vi "StanfordResSysDG645DelayGenerator.vi"() -> ()   [LabVIEW 2020]
uses:
  lib/Hardware/TextControlledInstrumIOQueuePacket.ctl
  lib/Hardware/TextControlledInstrum/TextControlledInstrumControlToCommandMulti.vi
panel:
  in  "SHOW LOG":bool
  in  "BURST":T1 {"Period (s)" format="%#_6p"; "Delay (s)" format="%#_6p"}
  in  "ErrChk":bool
  in  "Enable":bool
  out "ID":string
  in  "TRIGGER":T2 {"Level (V)" format="%#_6p"; "Rate (Hz)" format="%#_6p"; "Source" items=["Internal", "Ext Rising Edge", "Ext Falling Edge", "Single Shot Ext Rising", "Single Shot Ext Falling", "Single Shot", "Line"]}
  out "LOG":string
  in  "T0T1":T3 {"Delay T1" format="%#_6p"; "Delay T0" format="%#_6p"}
  in  "GH":T4 {"Delay H" format="%#_6p"; "Delay G" format="%#_6p"}
  in  "EF":T5 {"Delay F" format="%#_6p"; "Delay E" format="%#_6p"}
  in  "CD":T6 {"Delay D" format="%#_6p"; "Delay C" format="%#_6p"}
  in  "AB":T7 {"Delay B" format="%#_6p"; "Delay A" format="%#_6p"}
  in  "VISA resource name":refnum<visa-resource-name>
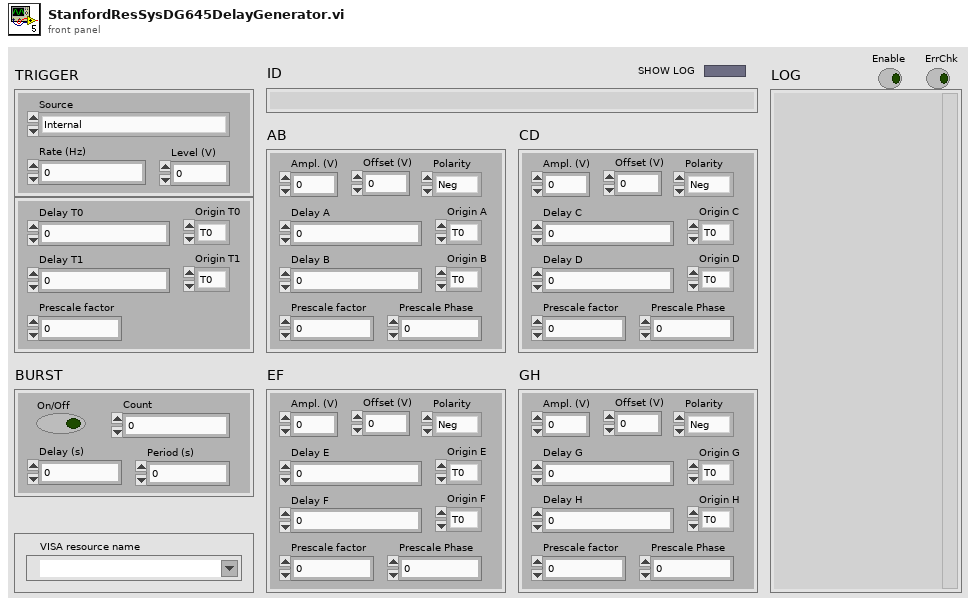
[diagram p1: front panel]
types:
  T1 = cluster{"On/Off":bool, "Count":u32, "Delay (s)":ext, "Period (s)":ext}
  T2 = cluster{"Source":u16, "Rate (Hz)":ext, "Level (V)":ext}
  T3 = cluster{"DLAY T0":string, "DLAY T1":string, "Delay T0":ext, "Origin T0":enum16{"T0", "T1", "A", "B", "C", "D", "E", "F", "G", "H"}, "Delay T1":ext, "Origin T1":enum16{"T0", "T1", "A", "B", "C", "D", "E", "F", "G", "H"}, "Prescale factor":u32}
  T4 = cluster{"Ampl. (V)":dbl, "Offset (V)":dbl, "Polarity":enum16{"Neg", "Pos"}, "DLAY G":string, "DLAY H":string, "Delay G":ext, "Origin G":enum16{"T0", "T1", "A", "B", "C", "D", "E", "F", "G", "H"}, "Delay H":ext, "Origin H":enum16{"T0", "T1", "A", "B", "C", "D", "E", "F", "G", "H"}, "Prescale factor":u32, "Prescale Phase":u32}
  T5 = cluster{"Ampl. (V)":dbl, "Offset (V)":dbl, "Polarity":enum16{"Neg", "Pos"}, "DLAY E":string, "DLAY F":string, "Delay E":ext, "Origin E":enum16{"T0", "T1", "A", "B", "C", "D", "E", "F", "G", "H"}, "Delay F":ext, "Origin F":enum16{"T0", "T1", "A", "B", "C", "D", "E", "F", "G", "H"}, "Prescale factor":u32, "Prescale Phase":u32}
  T6 = cluster{"Ampl. (V)":dbl, "Offset (V)":dbl, "Polarity":enum16{"Neg", "Pos"}, "DLAY C":string, "DLAY D":string, "Delay C":ext, "Origin C":enum16{"T0", "T1", "A", "B", "C", "D", "E", "F", "G", "H"}, "Delay D":ext, "Origin D":enum16{"T0", "T1", "A", "B", "C", "D", "E", "F", "G", "H"}, "Prescale factor":u32, "Prescale Phase":u32}
  T7 = cluster{"Ampl. (V)":dbl, "Offset (V)":dbl, "Polarity":enum16{"Neg", "Pos"}, "DLAY A":string, "DLAY B":string, "Delay A":ext, "Origin A":enum16{"T0", "T1", "A", "B", "C", "D", "E", "F", "G", "H"}, "Delay B":ext, "Origin B":enum16{"T0", "T1", "A", "B", "C", "D", "E", "F", "G", "H"}, "Prescale factor":u32, "Prescale Phase":u32}
  T8 = typedef "TextControlledInstrumIOQueuePacket.ctl" = cluster{"Operation":enum16{"read", "write", "reserved2", "reserved3", "reserved4", "reserved5", "reserved6", "reserved7"}, "Data":string, "Queue":refnum<queue>}
  T9 = enum16{"read", "write", "reserved2", "reserved3", "reserved4", "reserved5", "reserved6", "reserved7"}
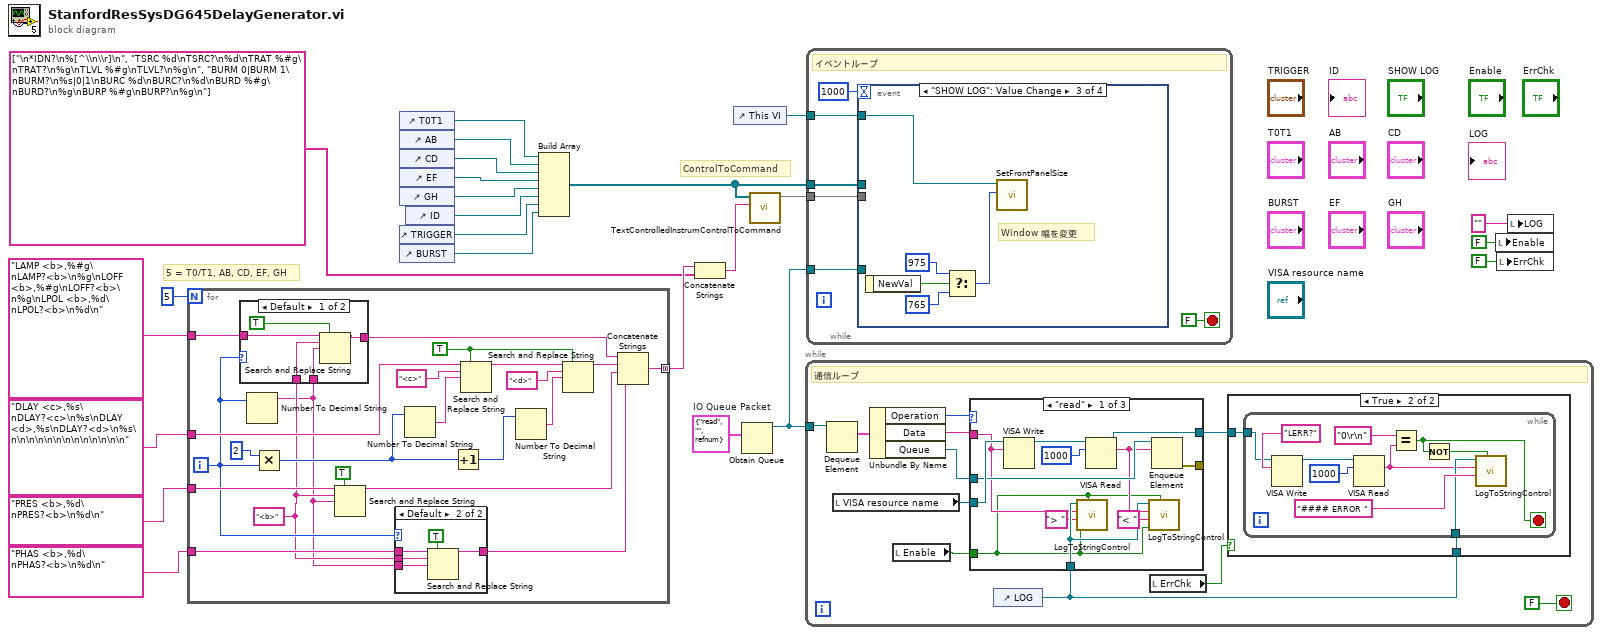
[diagram p0: block diagram]
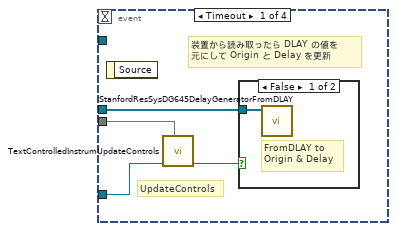
[diagram p4: hidden frame]
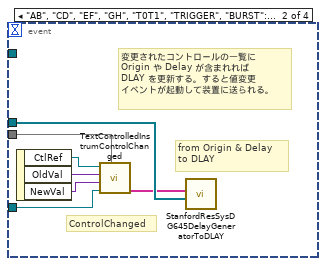
[diagram p6: hidden frame]
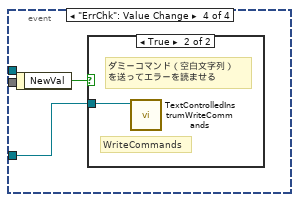
[diagram p7: hidden frame]
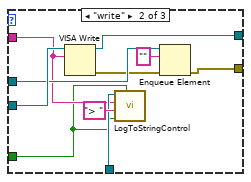
[diagram p9: hidden frame]
diagram:
  w15 = T8 {"Operation"=enum."read", "Data"="", "Queue"=refnum}  # IO Queue Packet
  # "ControlToCommand"
  # "5 = T0/T1, AB, CD, EF, GH"
  n1 = for {
    N: 5 -> [_]
    tunnel: "LAMP <b>,%#g\nLAMP?<b>\n%g\nLOFF <b>,%#g\nLOFF?<b>\n%g\nLPOL <b>,%d\nLPOL?<b>\n%d\n" -> [w46]
    tunnel: "DLAY <c>,%s\nDLAY?<c>\n%s\nDLAY <d>,%s\nDLAY?<d>\n%s\n\n\n\n\n\n\n\n\n\n\n\n\n" -> [w42]
    tunnel: [w34] -> w16 mode=concatenating
    tunnel: "PRES <b>,%d\nPRES?<b>\n%d\n" -> [w30]
    tunnel: "PHAS <b>,%d\nPHAS?<b>\n%d\n" -> [w29]
    i -> [w27]
    w26 = "<b>" ("search string")
    w33 = TRUE ("replace all? (F)")
    n2 = Number To Decimal String(number=w27) -> (decimal integer string=w25:string)  [unwired: 1 in]
    n3 = case shown="Default" w27 {
      tunnel: w46 -> [w56 _]
      tunnel: [w55 _] -> w35
      tunnel: w25 -> [w53 _]
      tunnel: w26 -> [w52 _]
      frame Default {
        n4 = Search and Replace String(replace all?=TRUE ("replace all? (F)"), input string=w56, search string=w52, replace string=w53) -> (result string=w55:string)  [unwired: 4 in, 3 out]
      }
      frame 0 {
      }
    }
    n5 = Multiply(x=2, y=w27) -> (x*y=w38:i32)
    n6 = Search and Replace String(replace all?=TRUE ("replace all? (F)"), input string=w30, search string=w26, replace string=w25) -> (result string=w31:string)  [unwired: 4 in, 3 out]
    n7 = case shown="Default" w27 {
      tunnel: w26 -> [_ w50]
      tunnel: w29 -> [_ w49]
      tunnel: [_ w48] -> w28
      tunnel: w25 -> [_ w47]
      frame 0 {
      }
      frame Default {
        n8 = Search and Replace String(replace all?=TRUE ("replace all? (F)"), input string=w49, search string=w50, replace string=w47) -> (result string=w48:string)  [unwired: 4 in, 3 out]
      }
    }
    n9 = Number To Decimal String(number=w38) -> (decimal integer string=w44:string)  [unwired: 1 in]
    n10 = Increment(x=w38) -> (x+1=w37:i32)
    n11 = Search and Replace String(replace all?=w33, input string=w42, search string="<c>", replace string=w44) -> (result string=w39:string)  [unwired: 4 in, 3 out]
    n12 = Number To Decimal String(number=w37) -> (decimal integer string=w41:string)  [unwired: 1 in]
    n13 = Search and Replace String(replace all?=w33, input string=w39, search string="<d>", replace string=w41) -> (result string=w36:string)  [unwired: 4 in, 3 out]
    n14 = Concatenate Strings(w35, w36, w31, w28) -> (w34:string)
  }
  n15 = control-ref of="T0T1"() -> (w24:refnum<vi>)
  n16 = control-ref of="AB"() -> (w23:refnum<vi>)
  n17 = control-ref of="CD"() -> (w22:refnum<vi>)
  n18 = control-ref of="EF"() -> (w21:refnum<vi>)
  n19 = control-ref of="GH"() -> (w20:refnum<vi>)
  n20 = control-ref of="TRIGGER"() -> (w10:refnum<vi>)
  n21 = control-ref of="BURST"() -> (w8:refnum<vi>)
  n22 = control-ref of="ID"() -> (w11:refnum<vi>)
  n23 = Build Array(w24, w23, w22, w21, w20, w11, w10, w8) -> (w2:refnum<vi>[])
  n24 = Concatenate Strings(w16, string[] ["\n*IDN?\n%[^\\n\\r]\n", "TSRC %d\nTSRC?\n%d\nTRAT %#g\nTRAT?\n%g\nTLVL %#g\nTLVL?\n%g\n", "BURM 0|BURM 1\nBURM?\n%s|0|1\nBURC %d\nBURC?\n%d\nBURD %#g\nBURD?\n%g\nBURP %#g\nBURP?\n%g\n"]) -> (w12:string)
  n25 = control-ref of="This VI"() -> (w5:refnum<vi>)
  n26 = Obtain Queue(element data type=w15) -> (queue out=w13:refnum<queue>)  [unwired: 4 in, 2 out]
  n27 = call-poly "TextControlledInstrumControlToCommand.vi"("SetGetCommands"=w12, "Control Array"=w2) -> ("ControlToCommand"=w14:map{refnum<vi>, string[]})  [unwired: 9 in]
  n28 = while {
    tunnel: w13 -> [w67]
    stop <- FALSE stop-if-true
    # "通信ループ"
    n29 = Dequeue Element(queue=w67) -> (element=w66:T8)  [unwired: 2 in, 3 out]
    n30 = local read "VISA resource name"() -> (w61:refnum<visa-resource-name>)
    n31 = Unbundle By Name(w66) -> ("Operation"=w65:T9, "Data"=w64:string, "Queue"=w63:refnum<queue>)
    n32 = local read "Enable"() -> (w58:bool)
    n33 = control-ref of="LOG"() -> (w59:refnum<vi>)
    n34 = case shown="\"read\"" w65 {
      tunnel: w64 -> [w73 w83 _]
      tunnel: w61 -> [w77 w89 w90]
      tunnel: w63 -> [w76 w88 _]
      tunnel: w59 -> [w75 w84 _]
      tunnel: [w70 w82 _] -> _
      tunnel: [w69 w81 w90] -> w60
      tunnel: w58 -> [w68 w80 _]
      frame "read" {
        n35 = VISA Write(VISA resource name=w77, write buffer=w73) -> (VISA resource name out=w79:refnum<visa-resource-name>)  [unwired: 1 in, 2 out]
        n36 = call "LogToStringControl.vi"("Enable"=w68, "Time Stamp (T/F or Format)"=w68, "Prefix (\"\")"="> " ("Prefix (\"\")"), "Log Text (\"\")"=w73, "String Ref"=w75) -> ()  [unwired: 6 in, 1 out]
        n37 = VISA Read(VISA resource name=w79, byte count=u32 1000) -> (VISA resource name out=w69:refnum<visa-resource-name>, read buffer=w74:string)  [unwired: 1 in, 2 out]
        n38 = call "LogToStringControl.vi"("Enable"=w68, "Time Stamp (T/F or Format)"=w68, "Prefix (\"\")"="< " ("Prefix (\"\")"), "Log Text (\"\")"=w74, "String Ref"=w75) -> ()  [unwired: 6 in, 1 out]
        n39 = Enqueue Element(queue=w76, element=w74) -> (error out=w70:errorcluster)  [unwired: 2 in, 2 out]
      }
      frame "write" {
        n40 = VISA Write(VISA resource name=w89, write buffer=w83) -> (VISA resource name out=w81:refnum<visa-resource-name>, error out=w86:errorcluster)  [unwired: 1 in, 1 out]
        n41 = call "LogToStringControl.vi"("Enable"=w80, "Time Stamp (T/F or Format)"=w80, "Prefix (\"\")"="> " ("Prefix (\"\")"), "Log Text (\"\")"=w83, "String Ref"=w84) -> ()  [unwired: 6 in, 1 out]
        n42 = Enqueue Element(queue=w88, element="", error in (no error)=w86) -> (error out=w82:errorcluster)  [unwired: 1 in, 2 out]
      }
      frame Default {
      }
    }
    n43 = local read "ErrChk"() -> (w57:bool)
    n44 = case shown="True" w57 {
      tunnel: w60 -> [_ w92]
      tunnel: w59 -> [_ w91]
      frame False {
      }
      frame True {
        n45 = while {
          tunnel: w92 -> [w99]
          tunnel: w91 -> [w97]
          stop <- w94 stop-if-true
          n46 = VISA Write(VISA resource name=w99, write buffer="LERR?") -> (VISA resource name out=w102:refnum<visa-resource-name>)  [unwired: 1 in, 2 out]
          n47 = VISA Read(VISA resource name=w102, byte count=u32 1000) -> (read buffer=w95:string)  [unwired: 1 in, 3 out]
          n48 = Equal?(x="0\r\n", y=w95) -> (x = y?=w94:bool)
          n49 = Not(x=w94) -> (.not. x?=w93:bool)
          n50 = call "LogToStringControl.vi"("Enable"=w93, "Prefix (\"\")"="#### ERROR " ("Prefix (\"\")"), "Log Text (\"\")"=w95, "String Ref"=w97) -> ()  [unwired: 7 in, 1 out]
        }
      }
    }
  }
  n51 = while {
    tunnel: w14 -> [w106]
    tunnel: w13 -> [w105]
    tunnel: w2 -> [w104]
    tunnel: w5 -> [w103]
    stop <- FALSE stop-if-true
    # "イベントループ"
    n52 = event shown="[2] \"SHOW LOG\": Value Change" {
      selector: _ -> [_ _ _ _]
      dyn-events: _ -> [_ _ _ _]
      timeout: 1000 -> [_ _ _ _]
      tunnel: w106 -> [w112 w117 _ _]
      tunnel: w105 -> [w109 w115 _ w126]
      tunnel: w104 -> [w110 w116 _ _]
      tunnel: w103 -> [_ _ w122 _]
      event Timeout {
        # "装置から読み取ったら DLAY の値を\n元にして Origin と Delay を更新"
        # "UpdateControls"
        n53 = event-data() -> ()  [unwired: 1 in, 1 out]
        n54 = call "TextControlledInstrumUpdateControls.vi"("ControlToCommand"=w112, "IO Queue"=w109) -> ("timed out?"=w111:bool)  [unwired: 9 in]
        n55 = case shown="False" w111 {
          tunnel: w110 -> [w113 _]
          frame False {
            # "FromDLAY to\nOrigin & Delay"
            n56 = call "StanfordResSysDG645DelayGeneratorFromDLAY.vi"("ControlArray"=w113) -> ()  [unwired: 11 in]
          }
          frame True {
          }
        }
      }
      event "AB", "CD", "EF", "GH", "T0T1", "TRIGGER", "BURST": Value Change {
        # "変更されたコントロールの一覧に\nOrigin や Delay が含まれれば\nDLAY を更新する。すると値変更\nイベントが起動して装置に送られる。"
        # "from Origin & Delay \nto DLAY"
        # "ControlChanged"
        n57 = event-data() -> ("CtlRef"=w120:refnum<vi>, "OldVal"=w119:variant, "NewVal"=w118:variant)  [unwired: 1 in]
        n58 = call "TextControlledInstrumControlChanged.vi"("ControlToCommand"=w117, "IO Queue"=w115, "NewVal"=w118, "OldVal"=w119, "CtlRef"=w120) -> ("Changed Names out"=w114:string[])  [unwired: 6 in]
        n59 = call "StanfordResSysDG645DelayGeneratorToDLAY.vi"("Control Array"=w116, "Changed Names in"=w114) -> ()  [unwired: 10 in]
      }
      event "SHOW LOG": Value Change {
        # "Window 幅を変更"
        n60 = event-data() -> ("NewVal"=w125:bool)  [unwired: 1 in]
        n61 = Select(t=u32 975 ("f"), s=w125, f=u32 765) -> (s? t:f=w121:u32)
        n62 = call "SetFrontPanelSize.vi"("Width (0: unchange)"=w121, "VI Reference"=w122) -> ()  [unwired: 9 in, 1 out]
      }
      event "ErrChk": Value Change {
        n63 = event-data() -> ("NewVal"=w127:bool)  [unwired: 1 in]
        n64 = case shown="True" w127 {
          tunnel: w126 -> [_ w128]
          frame False {
          }
          frame True {
            # "WriteCommands"
            # "ダミーコマンド（空白文字列）\nを送ってエラーを読ませる"
            n65 = call "TextControlledInstrumWriteCommands.vi"("IO Queue"=w128) -> ()  [unwired: 9 in, 2 out]
          }
        }
      }
    }
  }
  n66 = local write "Enable"(FALSE ("Enable")) -> ()
  n67 = local write "ErrChk"(FALSE ("ErrChk")) -> ()
  n68 = local write "LOG"("" ("ERROR LOG")) -> ()
